vi "get_response_headers.vi"(8 "error in (no error)":errorcluster, 11 "Request in":refnum<class "Request.lvclass">) -> (0 "error out":errorcluster, 2 "response_headers":refnum<class "Headers.lvclass">, 3 "Request in":refnum<class "Request.lvclass">)   [LabVIEW 2020, in "reqwest.lvlib" / "Request.lvclass"]
uses:
  Request.lvclass
  Headers/Headers.lvclass
  Request.lvclass/Request.ctl
  lv_reqwest_64.dll
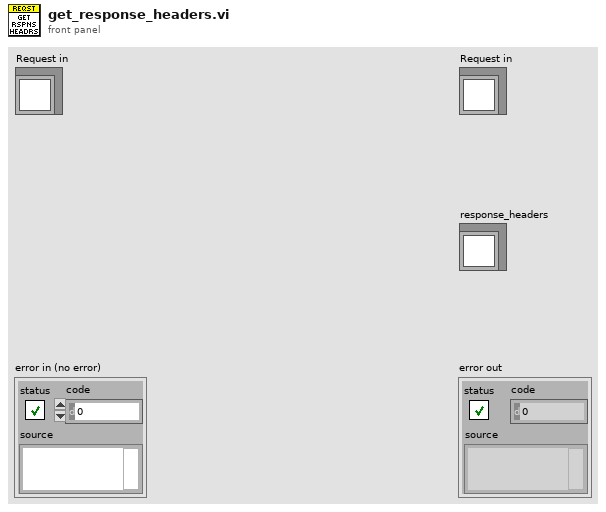
[diagram p1: front panel]
types:
  T1 = typedef "reqwest.lvlib/Request.lvclass/request_id.ctl" = u64
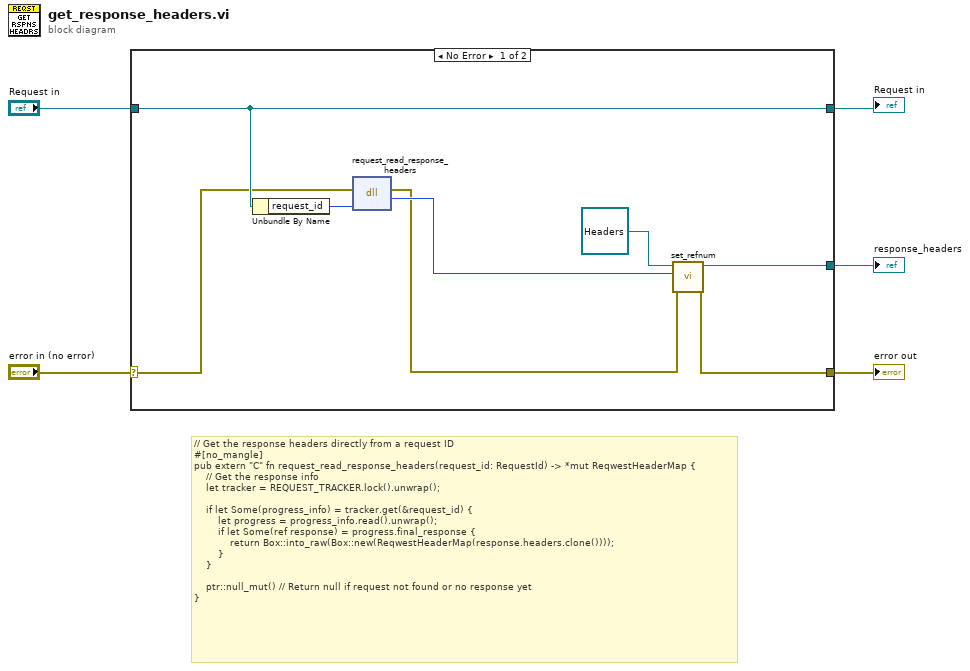
[diagram p0: block diagram]
diagram:
  # "// Get the response headers directly from a request ID\n#[no_mangle]\npub extern \"C\" fn request_read_response_headers(request_id: RequestId) -> *mut ReqwestHeaderMap {\n    // Get the response info\n    let tracker = REQUEST_TRACKER.lock().unwrap();\n    \n    if let Some(progress_info) = tracker.get(&request_id) {\n        let progress = progress_info.read().unwrap();\n        if let Some(ref response) = progress.final_response {\n            return Box::into_raw(Box::new(ReqwestHeaderMap(response.headers.clone())));\n        }\n    }\n    \n    ptr::null_mut() // Return null if request not found or no response yet\n}"
  n1 = case shown="No Error" "error in (no error)" {
    selector: "error in (no error)" -> [w11 w14]
    tunnel: "Request in" -> [w12 w15]
    tunnel: [w8 _] -> w1
    tunnel: [w7 w14] -> w2
    tunnel: [w12 w15] -> w3
    frame No Error {
      n2 = Unbundle By Name(w12) -> ("request_id"=w13:T1)
      n3 = dll-call lib="C:/Projects/reqwest-rs-labview/lv_src/lv_reqwest_*.*" fn="request_read_response_headers"(error in=w11, "request_id"=w13) -> (error out=w6:errorcluster, "headers_ptr"=w9:u64)  [unwired: 3 in, 1 out]
      n4 = call "set_refnum.vi"("error in (no error)"=w6, "ref"=w9, "Headers in"=refnum<class "Headers.lvclass"> refnum) -> ("error out"=w7:errorcluster, "Headers out"=w8:refnum<class "Headers.lvclass">)  [unwired: 7 in]
    }
    frame Error {
    }
  }
  "error out" <- w2
  "response_headers" <- w1
  "Request in" <- w3
